vi "Create.vi"(10 "Input":string) -> (1 "Parsed Array 2":string[](array[string]), 3 "Proto":refnum<class "Proto.lvclass">)   [LabVIEW 2020, in "Proto.lvclass"]
uses:
  Proto.lvclass
  Proto.lvclass/Proto.ctl
panel:
  out "Array":bool[](array[boolean])
  out "x+y":u64
  out "X":u64
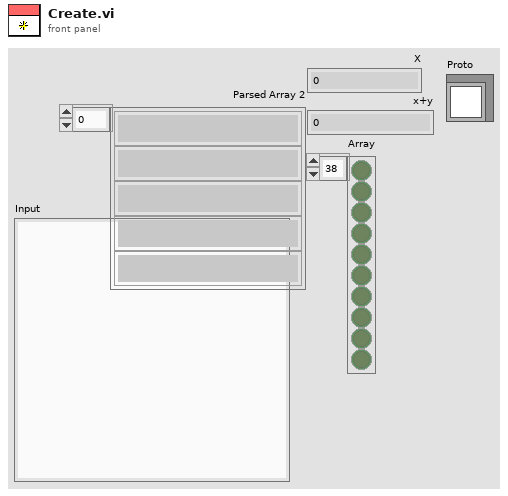
[diagram p1: front panel]
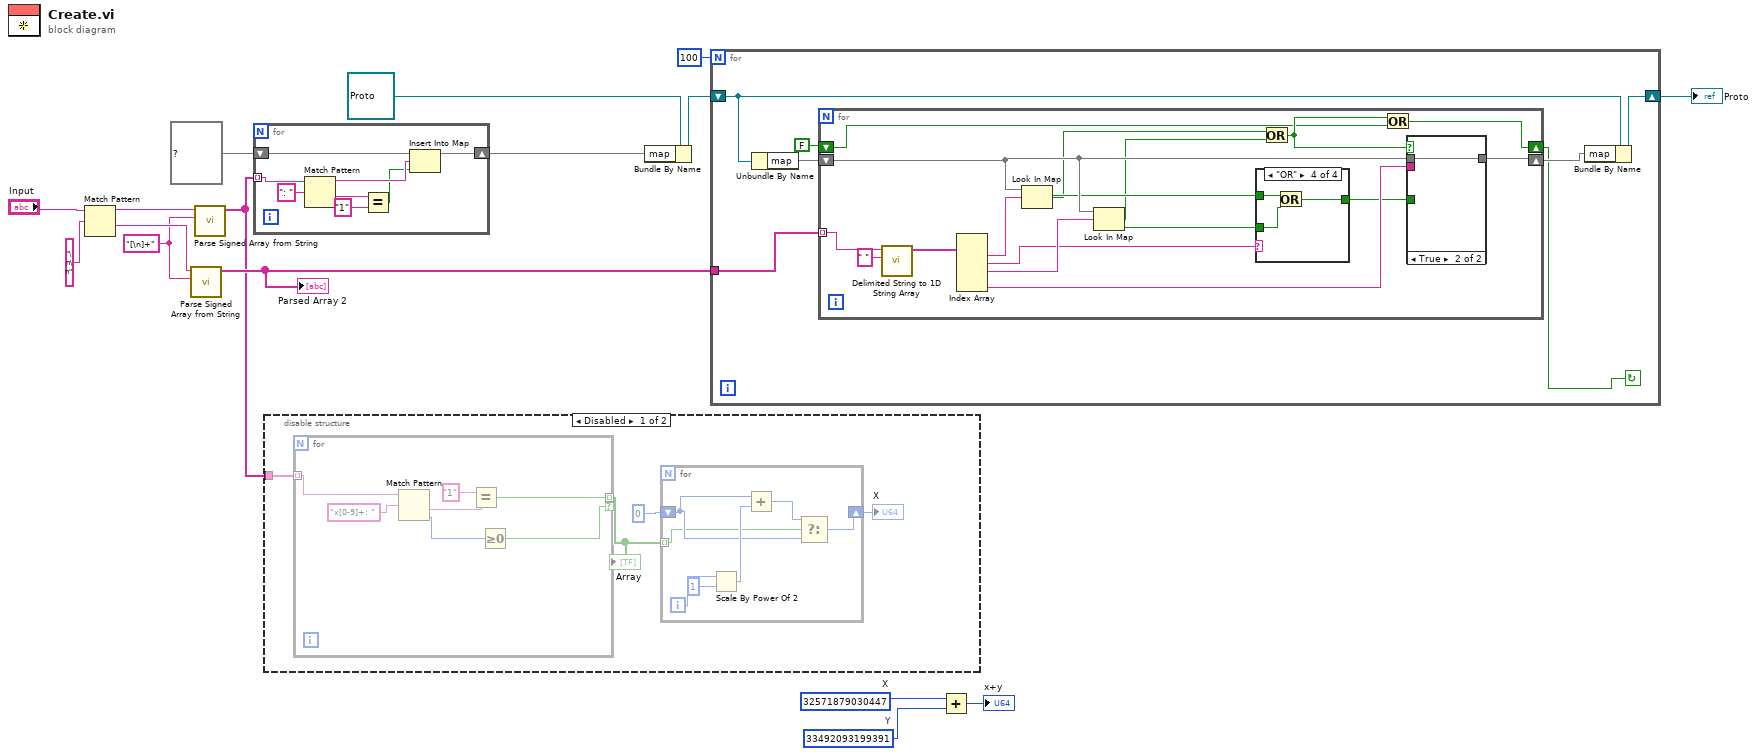
[diagram p0: block diagram]
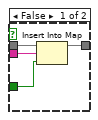
[diagram p2: hidden frame]
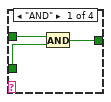
[diagram p3: hidden frame]
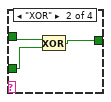
[diagram p4: hidden frame]
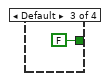
[diagram p5: hidden frame]
diagram:
  w4 = u64 33492093199391  # Y
  w5 = u64 32571879030447  # X
  w11 = "[\n]+" ("Delimiter regex")
  n1 = Match Pattern(string="Input", regular expression="\n\n") -> (before substring=w13:string, after substring=w12:string)  [unwired: 1 in, 2 out]
  n2 = call "Parse Signed Array from String.vi"("Delimiter regex"=w11, "Input"=w12) -> ("Parsed Array"=w7:string[])  [unwired: 8 in, 1 out]
  "Parsed Array 2" <- w7
  n3 = call "Parse Signed Array from String.vi"("Delimiter regex"=w11, "Input"=w13) -> ("Parsed Array"=w6:string[])  [unwired: 8 in, 1 out]
  n4 = for {
    tunnel: w6 -> [w22] mode=indexing
    shift-right: [w23] -> w9
    shift-left: map{string, bool} {} ("map") -> [w24]
    n5 = Match Pattern(string=w22, regular expression=": ") -> (before substring=w20:string, after substring=w19:string)  [unwired: 1 in, 2 out]
    n6 = Equal?(x=w19, y="1") -> (x = y?=w17:bool)
    n7 = Insert Into Map(map in=w24, key=w20, value=w17) -> (map out=w23:map{string, bool})  [unwired: 2 out]
  }
  n8 = disable-structure shown="Disabled" {
    disable-tunnel: w6 -> [w28 _]
    frame Disabled {
      n9 = for {
        tunnel: w28 -> [w39] mode=indexing
        tunnel: [w40] -> w27 mode=indexing if=w36
        n10 = Match Pattern(string=w39, regular expression="x[0-9]+: " ("string")) -> (after substring=w42:string, offset past match=w37:i32)  [unwired: 1 in, 2 out]
        n11 = Equal?(x="1", y=w42) -> (x = y?=w40:bool)
        n12 = Greater Or Equal To 0?(x=w37) -> (x >= 0?=w36:bool)
      }
      "Array" <- w27
      n13 = for {
        tunnel: w27 -> [w31] mode=indexing
        shift-right: [w29] -> w25
        shift-left: u64 0 ("number") -> [w32]
        i -> [w35]
        n14 = Scale By Power Of 2(n=w35, x=u64 1) -> (x*2^n=w33:u64)
        n15 = Add(x=w32, y=w33) -> (x+y=w30:u64)
        n16 = Select(t=w30, s=w31, f=w32) -> (s? t:f=w29:u64)
      }
      "X" <- w25
    }
    frame Enabled {
    }
  }
  n17 = Bundle By Name(cluster=refnum<class "Proto.lvclass"> refnum ("Proto"), "map"=w9) -> (w8:refnum<class "Proto.lvclass">)
  n18 = for {
    N: 100 -> [_]
    tunnel: w7 -> [w47]
    shift-right: [w46] -> w2
    shift-left: w8 -> [w49]
    stop <- w43 continue-if-true
    n19 = Unbundle By Name(w49) -> ("map"=w48:map{string, bool})
    n20 = for {
      shift-right: [w66] -> w45
      shift-left: w48 -> [w65]
      tunnel: w47 -> [w64] mode=indexing
      shift-right: [w51] -> w43
      shift-left: FALSE -> [w50]
      n21 = call <vilib>:"Delimited String to 1D String Array.vi"("delimiter"=" ", "delimited string"=w64) -> ("string array"=w62:string[])  [unwired: 9 in]
      n22 = Index Array(array=w62) -> (element #1=w60:string, element #2=w58:string, element #3=w59:string, element #5=w61:string)  [unwired: 5 in, 1 out]
      n23 = Look In Map(map=w65, key=w60) -> (key not found?=w53:bool, value=w57:bool)  [unwired: 1 in]
      n24 = Look In Map(map=w65, key=w59) -> (key not found?=w54:bool, value=w56:bool)  [unwired: 1 in]
      n25 = case shown="\"OR\"" w58 {
        tunnel: w57 -> [w74 w77 _ w81]
        tunnel: w56 -> [w73 w76 _ w80]
        tunnel: [w72 w75 FALSE w79] -> w55
        frame "AND" {
          n26 = And(x=w74, y=w73) -> (x .and. y?=w72:bool)
        }
        frame "XOR" {
          n27 = Exclusive Or(1:w76, 2:w77) -> (0:w75:bool)
        }
        frame Default {
        }
        frame "OR" {
          n28 = Or(x=w81, y=w80) -> (x .or. y?=w79:bool)
        }
      }
      n29 = Or(x=w53, y=w54) -> (x .or. y?=w52:bool)
      n30 = Or(x=w52, y=w50) -> (x .or. y?=w51:bool)
      n31 = case shown="True" w52 {
        tunnel: [w70 w71] -> w66
        tunnel: w65 -> [w69 w71]
        tunnel: w61 -> [w68 _]
        tunnel: w55 -> [w67 _]
        frame False {
          n32 = Insert Into Map(map in=w69, key=w68, value=w67) -> (map out=w70:map{string, bool})  [unwired: 2 out]
        }
        frame True {
        }
      }
    }
    n33 = Bundle By Name(cluster=w49, "map"=w45) -> (w46:refnum<class "Proto.lvclass">)
  }
  "Proto" <- w2
  n34 = Add(x=w5, y=w4) -> (x+y=→"x+y":u64)
